vi "Relink.vi"(0 "Executioner in":refnum<class "Executioner.lvclass">, 1 "Linked List Ref":refnum<data-value>, 2 "File Path":path, 5 "Flattened Test Executive":string, 7 "Return":string, 9 "Linked List ID":string, 11 "error in (no error)":errorcluster, 12 "Persistence in":refnum<class "IPersist.lvclass">, 13 "Compatibility Helper":refnum<class "ICompatibility Helper.lvclass">, 14 "Path Builder":refnum<class "IPath Builder.lvclass">) -> (3 "Linked List Ref out":refnum<data-value>, 6 "Flattened Test Executive out":string, 8 "Return out":string, 15 "error out":errorcluster)   [LabVIEW 2020, in "Test Executive.lvlib" / "Executioner.lvclass"]
uses:
  <vilib>/gpm_packages/@cs/test-executive/Source/Test Executive/Executioner/Executioner.lvclass
  <vilib>/gpm_packages/@cs/persistence/source/IPersist/IPersist.lvclass
  <vilib>/gpm_packages/@cs/linked-list/Source/Linked List/ILinkedList/ILinked List.lvclass
  <vilib>/gpm_packages/@cs/test-executive/Source/Path Builder/IPath Builder/IPath Builder.lvclass
  <vilib>/gpm_packages/@cs/test-executive/Source/Compatibility Helper/ICompatibility Helper.lvclass
  7496b3ab-09a6-44dc-ae9e-1065b628b99e.vi
  <vilib>/Utility/error.llb/Error Cluster From Error Code.vi
  <vilib>/ErrorRing/Error Ring.xnode
  <vilib>/gpm_packages/@cs/linked-list/Source/Linked List/Linked List Ref/Linked List Ref.lvclass
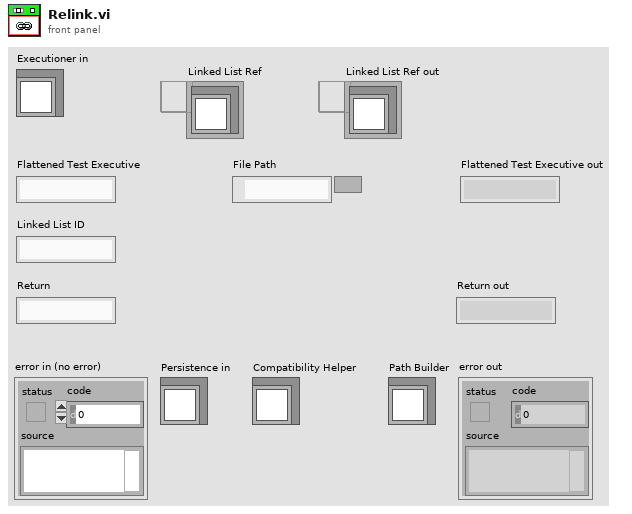
[diagram p1: front panel]
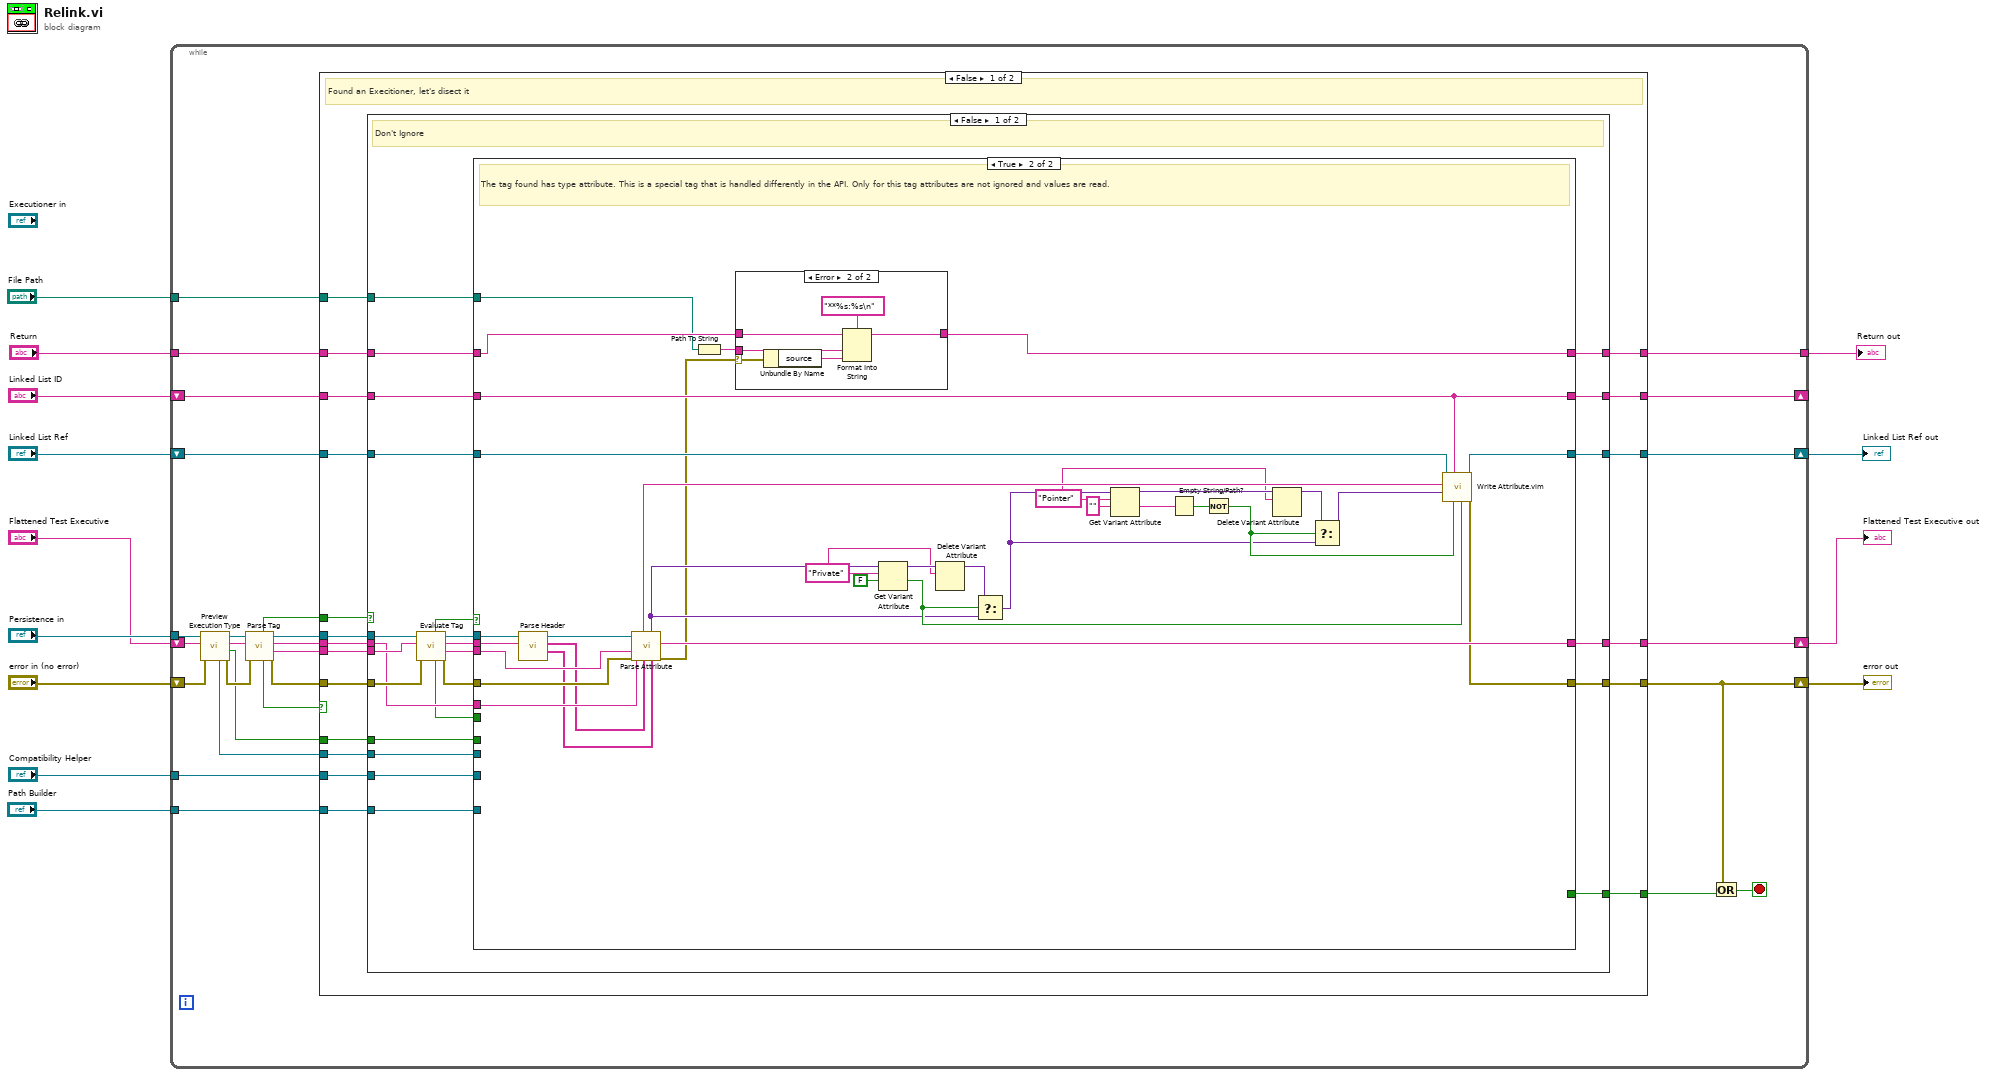
[diagram p0: block diagram]
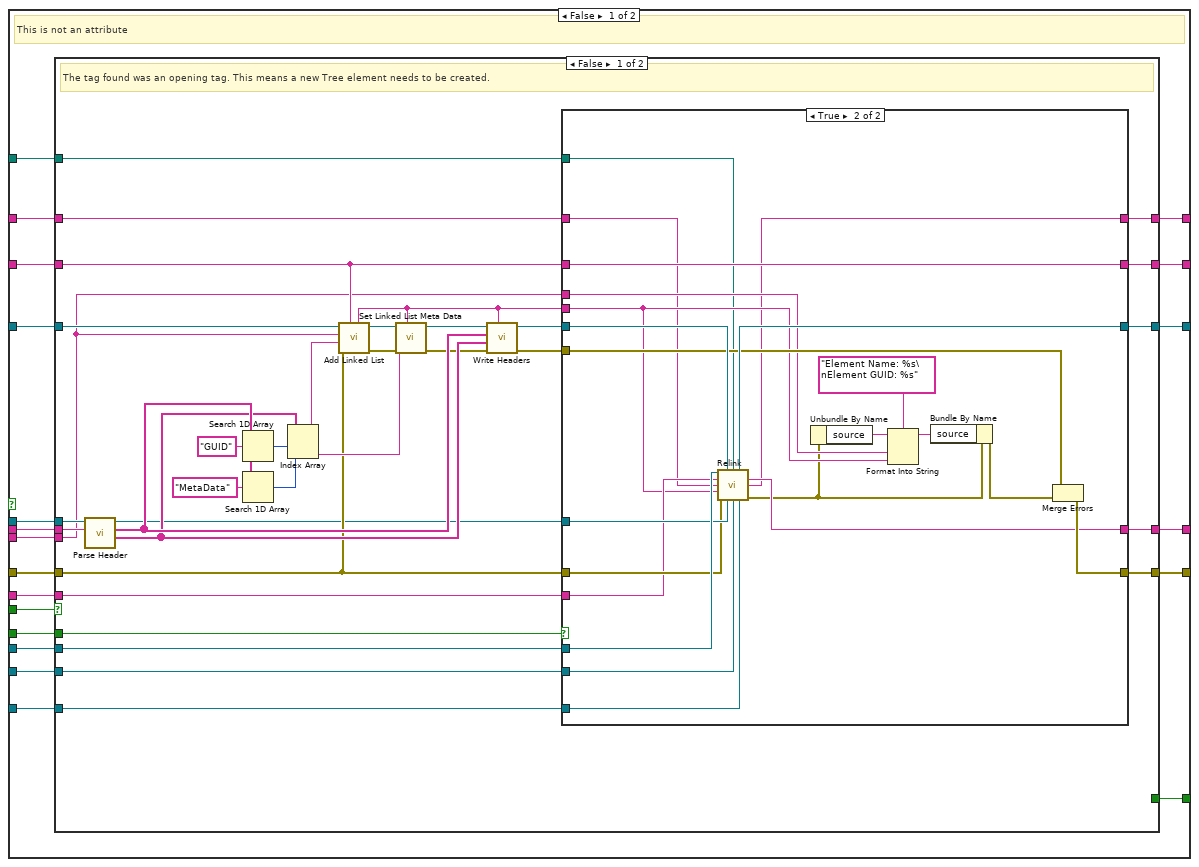
[diagram p2: hidden frame]
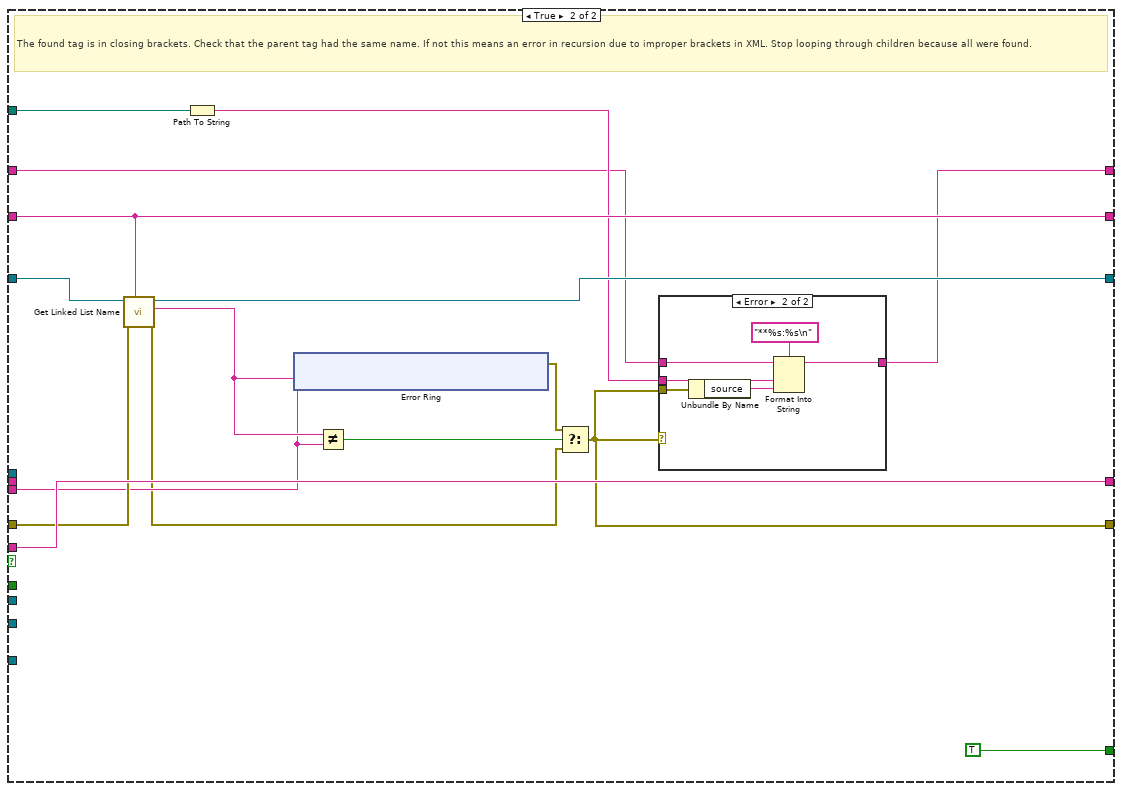
[diagram p4: hidden frame]
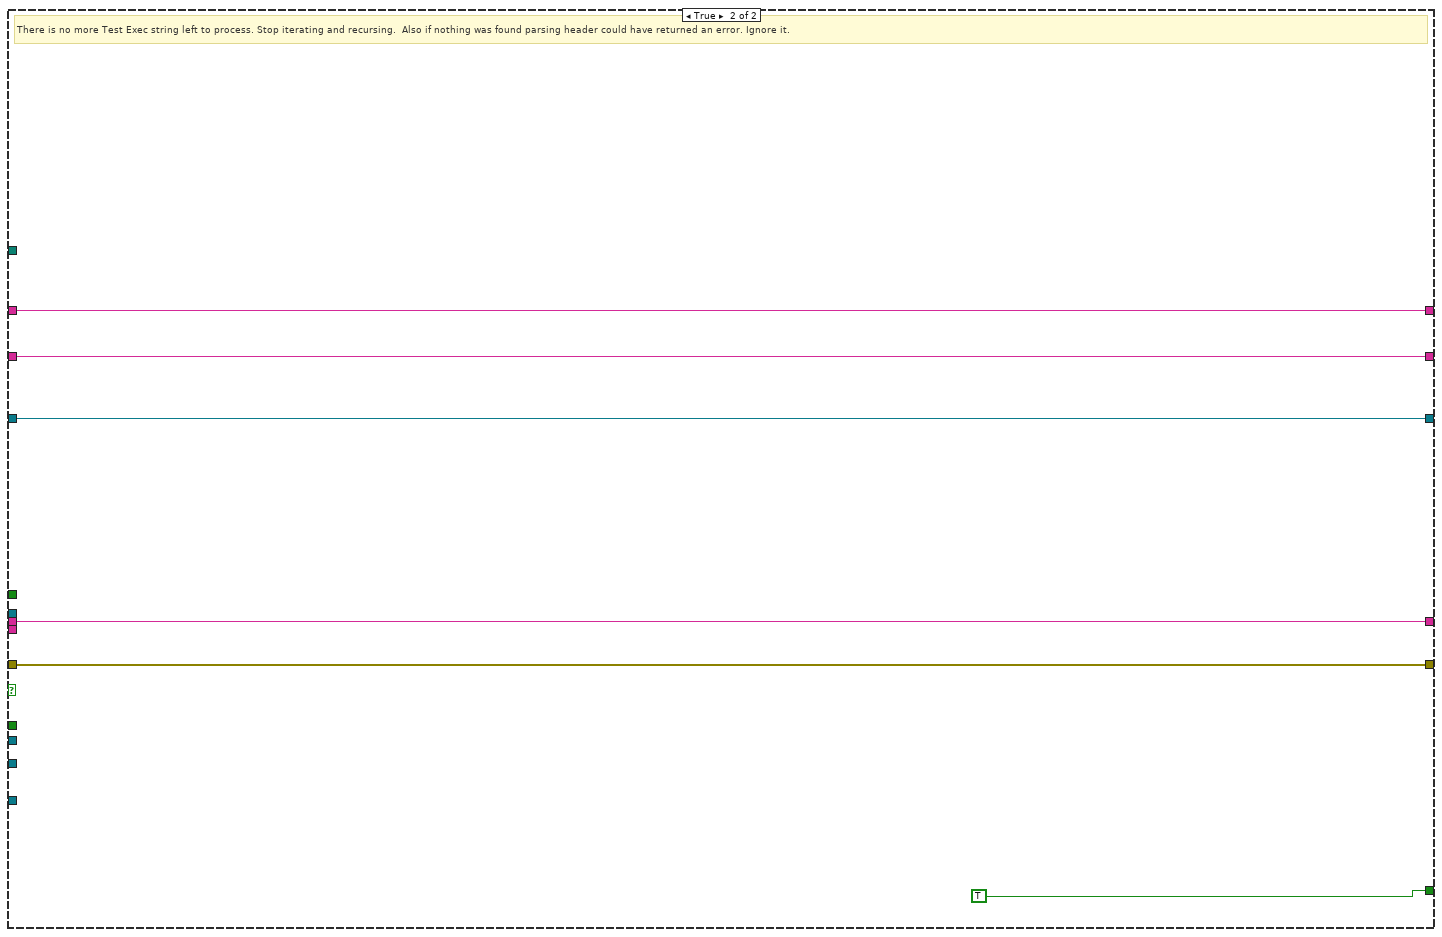
[diagram p8: hidden frame]
diagram:
  n1 = while {
    shift-right: [w38] -> w6
    shift-left: "Flattened Test Executive" -> [w32]
    shift-right: [w17] -> w10
    shift-left: "Linked List Ref" -> [w40]
    shift-right: [w36] -> w7
    shift-left: "error in (no error)" -> [w30]
    shift-right: [w20] -> _
    shift-left: "Linked List ID" -> [w35]
    tunnel: "Persistence in" -> [w34]
    tunnel: "Path Builder" -> [w19]
    tunnel: "Compatibility Helper" -> [w18]
    tunnel: "File Path" -> [w16]
    tunnel: "Return" -> [w15]
    tunnel: [w14] -> w1
    stop <- w37 stop-if-true
    n2 = call <vilib>:"Preview Execution Type.vi"("error in (no error)"=w30, "Flattened Linked List"=w32, "IPersist in"=w34) -> ("error out"=w29:errorcluster, "Found?"=w22:bool, "Flattened Linked List out"=w31:string, "IPersist out"=w33:refnum<class "IPersist.lvclass">, "Execution Type"=w21:refnum<class "Executioner.lvclass">)  [unwired: 4 in]
    n3 = call-dynamic "Parse Tag.vi"("error in (no error)"=w29, "Flattened Linked List"=w31, "IPersist in"=w33) -> ("error out"=w24:errorcluster, "Tag"=w26:string, "Flattened Linked List After Tag"=w25:string, "IPersist out"=w27:refnum<class "IPersist.lvclass">, "Nothing Found"=w23:bool, "Ignore"=w28:bool)  [unwired: 2 in, 1 out]
    n4 = case shown="False" w23 {
      tunnel: w27 -> [w56 _]
      tunnel: w26 -> [w50 _]
      tunnel: w25 -> [w55 w245]
      tunnel: w24 -> [w52 w244]
      tunnel: w28 -> [w59 _]
      tunnel: w22 -> [w48 _]
      tunnel: w35 -> [w49 w243]
      tunnel: w40 -> [w58 w247]
      tunnel: [w57 w247] -> w17
      tunnel: [w51 TRUE] -> w39
      tunnel: [w54 w245] -> w38
      tunnel: [w53 w244] -> w36
      tunnel: w21 -> [w47 _]
      tunnel: [w46 w243] -> w20
      tunnel: w19 -> [w45 _]
      tunnel: w18 -> [w44 _]
      tunnel: w16 -> [w43 _]
      tunnel: w15 -> [w42 w242]
      tunnel: [w41 w242] -> w14
      frame False {
        # "Found an Execitioner, let's disect it"
        n5 = case shown="False" w59 {
          tunnel: w58 -> [w76 w241]
          tunnel: [w68 w241] -> w57
          tunnel: w56 -> [w83 _]
          tunnel: w55 -> [w74 w240]
          tunnel: [w69 w240] -> w54
          tunnel: [w79 w239] -> w53
          tunnel: w52 -> [w81 w239]
          tunnel: [w67 _] -> w51
          tunnel: w50 -> [w82 _]
          tunnel: w49 -> [w75 w238]
          tunnel: w48 -> [w73 _]
          tunnel: w47 -> [w66 _]
          tunnel: [w65 w238] -> w46
          tunnel: w45 -> [w64 _]
          tunnel: w44 -> [w63 _]
          tunnel: w43 -> [w62 _]
          tunnel: w42 -> [w61 w237]
          tunnel: [w60 w237] -> w41
          frame False {
            # "Don't Ignore"
            n6 = call-dynamic "Evaluate Tag.vi"("error in (no error)"=w81, "Tag"=w82, "IPersist in"=w83) -> ("error out"=w80:errorcluster, "Tag Name"=w71:string, "Header"=w72:string, "IPersist out"=w77:refnum<class "IPersist.lvclass">, "End of Tag"=w70:bool, "Attribute"=w78:bool)  [unwired: 3 in]
            n7 = case shown="True" w78 {
              tunnel: w80 -> [w98 w224]
              tunnel: [w94 w210] -> w79
              tunnel: w77 -> [w103 w229]
              tunnel: w76 -> [w101 w215]
              tunnel: w75 -> [w89 w209]
              tunnel: w74 -> [w97 w225]
              tunnel: w73 -> [w96 _]
              tunnel: w72 -> [w102 w228]
              tunnel: w71 -> [w99 w226]
              tunnel: w70 -> [w100 _]
              tunnel: [w93 w221] -> w69
              tunnel: [w95 w214] -> w68
              tunnel: [w92 _] -> w67
              tunnel: w66 -> [w91 _]
              tunnel: [w90 w209] -> w65
              tunnel: w64 -> [w88 _]
              tunnel: w63 -> [w87 _]
              tunnel: w62 -> [w86 w196]
              tunnel: w61 -> [w85 w199]
              tunnel: [w84 w198] -> w60
              frame False {
                # "This is not an attribute"
                n8 = case shown="False" w100 {
                  tunnel: w103 -> [w137 _]
                  tunnel: w102 -> [w136 _]
                  tunnel: w101 -> [w131 w179]
                  tunnel: w99 -> [w107 w173]
                  tunnel: w98 -> [w114 w176]
                  tunnel: w97 -> [w115 w178]
                  tunnel: w96 -> [w116 _]
                  tunnel: w89 -> [w110 w171]
                  tunnel: [w122 w177] -> w95
                  tunnel: [w118 w167] -> w94
                  tunnel: [w117 w178] -> w93
                  tunnel: [_ TRUE] -> w92
                  tunnel: w91 -> [w112 _]
                  tunnel: [w111 w171] -> w90
                  tunnel: w88 -> [w109 _]
                  tunnel: w87 -> [w108 _]
                  tunnel: w86 -> [w106 w169]
                  tunnel: w85 -> [w105 w166]
                  tunnel: [w104 w165] -> w84
                  frame False {
                    # "The tag found was an opening tag. This means a new Tree element needs to be created."
                    n9 = call-dynamic "Parse Header.vi"("Header"=w136, "IPersist in"=w137) -> ("Value"=w124:string[], "Name"=w125:string[], "IPersist out"=w113:refnum<class "IPersist.lvclass">)  [unwired: 7 in]
                    n10 = Search 1D Array(1D array=w125, element="GUID") -> (index of element=w133:i32)  [unwired: 1 in]
                    n11 = Search 1D Array(1D array=w125, element="MetaData") -> (index of element=w132:i32)  [unwired: 1 in]
                    n12 = Index Array(array=w124, index #1=w133, index #2=w132) -> (element #1=w130:string, element #2=w127:string)
                    n13 = call <vilib>:"Add Linked List.vi"("Parent ID"=w110, "error in (no error)"=w114, "Linked List ID"=w130, "Name"=w107, "Linked List Ref"=w131) -> ("error out"=w128:errorcluster, "Linked List Ref out"=w129:refnum<data-value>, "Linked List ID out"=w120:string)  [unwired: 3 in, 1 out]
                    n14 = call <vilib>:"Set Linked List Meta Data.vi"("Linked List ID"=w120, "error in (no error)"=w128, "Meta Data"=w127, "Linked List Ref"=w129) -> ("error out"=w123:errorcluster, "Linked List Ref out"=w126:refnum<data-value>)  [unwired: 5 in, 1 out]
                    n15 = call <vilib>:"Write Headers.vi"("Linked List ID"=w120, "error in (no error)"=w123, "Header Values"=w124, "Header Names"=w125, "Linked List Ref"=w126) -> ("error out"=w119:errorcluster, "Linked List Ref out"=w121:refnum<data-value>)  [unwired: 5 in]
                    n16 = case shown="True" w116 {
                      tunnel: [w142 w164] -> w122
                      tunnel: w121 -> [w142 w163]
                      tunnel: w120 -> [w139 w150]
                      tunnel: w119 -> [w141 w162]
                      tunnel: [w141 w161] -> w118
                      tunnel: [w140 w160] -> w117
                      tunnel: w113 -> [_ w158]
                      tunnel: w115 -> [w140 w156]
                      tunnel: w114 -> [_ w157]
                      tunnel: w112 -> [_ w159]
                      tunnel: w110 -> [_ w155]
                      tunnel: [w139 w155] -> w111
                      tunnel: w109 -> [_ w154]
                      tunnel: w108 -> [_ w153]
                      tunnel: w107 -> [_ w149]
                      tunnel: w106 -> [_ w145]
                      tunnel: w105 -> [w138 w144]
                      tunnel: [w138 w143] -> w104
                      frame False {
                      }
                      frame True {
                        n17 = call-dynamic "Relink.vi"("Executioner in"=w159, "Linked List Ref"=w163, "File Path"=w145, "Flattened Test Executive"=w156, "Return"=w144, "Linked List ID"=w150, "error in (no error)"=w157, "Persistence in"=w158, "Compatibility Helper"=w153, "Path Builder"=w154) -> ("Linked List Ref out"=w164:refnum<data-value>, "Flattened Test Executive out"=w160:string, "Return out"=w143:string, "error out"=w148:errorcluster)  [unwired: 2 in]
                        n18 = Unbundle By Name(w148) -> ("source"=w152:string)
                        n19 = Format Into String(format string="Element Name: %s\nElement GUID: %s", initial string=w152, w149, w150) -> (resulting string=w146:string)  [unwired: 1 in, 1 out]
                        n20 = Bundle By Name(cluster=w148, "source"=w146) -> (w147:errorcluster)
                        n21 = Merge Errors(w162, w147) -> (w161:errorcluster)
                      }
                    }
                  }
                  frame True {
                    # "The found tag is in closing brackets. Check that the parent tag had the same name. If not this means an error in recursion due to improper brackets in XML. Stop looping through children because all were found."
                    n22 = call <vilib>:"Get Linked List Name.vi"("Linked List ID"=w171, "error in (no error)"=w176, "Linked List Ref"=w179) -> ("error out"=w172:errorcluster, "Linked List Name"=w174:string, "Linked List Ref out"=w177:refnum<data-value>)  [unwired: 5 in, 1 out]
                    n23 = Path To String(path=w169) -> (string=w168:string)
                    n24 = xnode "Error Ring"("parameter 0"=w174, "parameter 1"=w173) -> ("error out"=w170:errorcluster)
                    n25 = Not Equal?(x=w174, y=w173) -> (x != y?=w175:bool)
                    n26 = Select(t=w170, s=w175, f=w172) -> (s? t:f=w167:errorcluster)
                    n27 = case shown="Error" w167 {
                      tunnel: w168 -> [_ w186]
                      tunnel: w167 -> [_ w185]
                      tunnel: w166 -> [w181 w183]
                      tunnel: [w181 w182] -> w165
                      frame No Error {
                      }
                      frame Error {
                        n28 = Unbundle By Name(w185) -> ("source"=w184:string)
                        n29 = Format Into String(format string="**%s:%s\n", initial string=w183, w186, w184) -> (resulting string=w182:string)  [unwired: 1 in, 1 out]
                      }
                    }
                  }
                }
              }
              frame True {
                w202 = "Private" ("name")
                w201 = "Pointer" ("name")
                # "The tag found has type attribute. This is a special tag that is handled differently in the API. Only for this tag attributes are not ignored and values are read."
                n30 = call-dynamic "Parse Header.vi"("Header"=w228, "IPersist in"=w229) -> ("Value"=w222:string[], "Name"=w223:string[], "IPersist out"=w227:refnum<class "IPersist.lvclass">)  [unwired: 7 in]
                n31 = call-dynamic "Parse Attribute.vi"("Header Values"=w222, "Header Names"=w223, "error in (no error)"=w224, "Tag Name"=w226, "Flattened Linked List"=w225, "IPersist in"=w227) -> ("error out"=w200:errorcluster, "Flattened Linked List out"=w221:string, "Attribute Value"=w204:variant, "Attribute Name"=w212:string)  [unwired: 1 in, 1 out]
                n32 = Path To String(path=w196) -> (string=w197:string)
                n33 = case shown="Error" w200 {
                  selector: w200 -> [_ w234]
                  tunnel: w197 -> [_ w235]
                  tunnel: w199 -> [w230 w232]
                  tunnel: [w230 w231] -> w198
                  frame No Error {
                  }
                  frame Error {
                    n34 = Unbundle By Name(w234) -> ("source"=w233:string)
                    n35 = Format Into String(format string="**%s:%s\n", initial string=w232, w235, w233) -> (resulting string=w231:string)  [unwired: 1 in, 1 out]
                  }
                }
                n36 = Get Variant Attribute(Variant=w204, name=w202, default value (empty Variant)=FALSE) -> (duplicate Variant=w207:variant, value=w205:bool)  [unwired: 1 in, 2 out]
                n37 = Delete Variant Attribute(6:w202, 7:w207) -> (3:w208:variant)  [unwired: 1 in, 2 out]
                n38 = Select(t=w208, s=w205, f=w204) -> (s? t:f=w203:variant)
                n39 = Get Variant Attribute(Variant=w203, name=w201, default value (empty Variant)="") -> (duplicate Variant=w219:variant, value=w217:string)  [unwired: 1 in, 2 out]
                n40 = Empty String/Path?(string/path=w217) -> (empty?=w216:bool)
                n41 = Not(x=w216) -> (.not. x?=w213:bool)
                n42 = Delete Variant Attribute(6:w201, 7:w219) -> (3:w218:variant)  [unwired: 1 in, 2 out]
                n43 = Select(t=w218, s=w213, f=w203) -> (s? t:f=w211:variant)
                n44 = call "Write Attribute.vim"("Private?"=w205, "Pointer?"=w213, "Linked List ID"=w209, "Attribute"=w211, "Attribute Name"=w212, "Linked List Ref"=w215) -> ("error out"=w210:errorcluster, "Linked List Ref out"=w214:refnum<data-value>)  [unwired: 2 in, 2 out]
              }
            }
          }
          frame True {
            # "Ignore this element due to syntax of header"
          }
        }
      }
      frame True {
        # "There is no more Test Exec string left to process. Stop iterating and recursing.  Also if nothing was found parsing header could have returned an error. Ignore it."
      }
    }
    n45 = Or(x=w36, y=w39) -> (x .or. y?=w37:bool)
  }
  "error out" <- w7
  "Flattened Test Executive out" <- w6
  "Linked List Ref out" <- w10
  "Return out" <- w1
